vi "BLAS1 Utility(CDB).vi"(0 "x":cdb[](array[numeric]), 1 "y":cdb[](array[numeric]), 2 "xInc":i32, 3 "yInc":i32, 6 "function":T1 items=["ddot/zdotu/zdotc", "daxpy/zaxpy", "dnrm2/dznrm2", "dasum/dzasum", "dcopy/zcopy", "dswap/zswap", "drotm", "drot/zdrot", "idamax/izamax", "idamin/izamin", "dgemv/zgemv", "dsymv/zhemv", "dtrmv/ztrmv", "dsyr/zher", "dsyr2/zher2", "dger/zgeru/zgerc", "dtrsv/ztrsv", "dgemm/zgemm", "dsymm/zsymm/zhemm", "dtrmm/ztrmm", "dsyrk/zsyrk/zherk", "dsyr2k/zsyr2k/zher2k", "dtrsm/ztrsm"]) -> (19 "n":i32)   [LabVIEW 2017, in "NI_AALBLAS.lvlib"]
uses:
  NI_AALBLAS.lvlib
  Fucntion.ctl
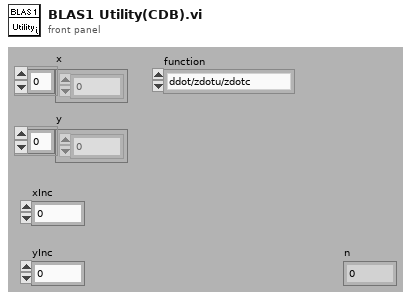
[diagram p1: front panel]
types:
  T1 = typedef "NI_AALBLAS.lvlib/Fucntion.ctl" = u16
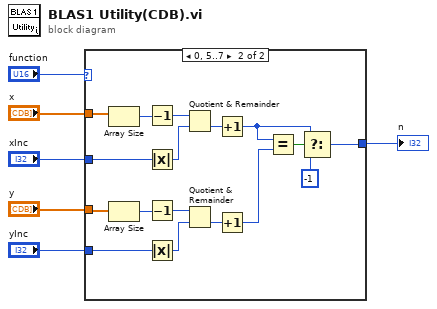
[diagram p0: block diagram]
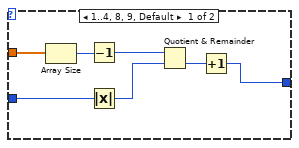
[diagram p2: hidden frame]
diagram:
  n1 = case shown="0, 5..7" "function" {
    tunnel: "x" -> [w13 w22]
    tunnel: "y" -> [_ w20]
    tunnel: [w9 w18] -> w4
    tunnel: "xInc" -> [w10 w21]
    tunnel: "yInc" -> [_ w19]
    frame 1..4, 8, 9, Default {
      n2 = Array Size(array=w13) -> (size(s)=w11:i32)
      n3 = Decrement(x=w11) -> (x-1=w8:i32)
      n4 = Absolute Value(x=w10) -> (abs(x)=w7:i32)
      n5 = Quotient & Remainder(x=w8, y=w7) -> (floor(x/y)=w12:i32)  [unwired: 1 out]
      n6 = Increment(x=w12) -> (x+1=w9:i32)
    }
    frame 0, 5..7 {
      n7 = Array Size(array=w22) -> (size(s)=w28:i32)
      n8 = Array Size(array=w20) -> (size(s)=w24:i32)
      n9 = Decrement(x=w28) -> (x-1=w17:i32)
      n10 = Absolute Value(x=w21) -> (abs(x)=w15:i32)
      n11 = Decrement(x=w24) -> (x-1=w16:i32)
      n12 = Absolute Value(x=w19) -> (abs(x)=w14:i32)
      n13 = Quotient & Remainder(x=w17, y=w15) -> (floor(x/y)=w27:i32)  [unwired: 1 out]
      n14 = Quotient & Remainder(x=w16, y=w14) -> (floor(x/y)=w25:i32)  [unwired: 1 out]
      n15 = Increment(x=w27) -> (x+1=w26:i32)
      n16 = Increment(x=w25) -> (x+1=w23:i32)
      n17 = Equal?(x=w26, y=w23) -> (x = y?=w30:bool)
      n18 = Select(t=w26, s=w30, f=-1) -> (s? t:f=w18:i32)
    }
  }
  "n" <- w4
